vi "NIFPGA-MCS.get scan status.vi"(0 "i ref in":refnum<vi>, 3 "ms timeout (10000)":i32=10000, 5 "error in (no error)":errorcluster) -> (14 "i ref out":refnum<vi>, 16 "scanFinished ?":bool, 17 "timed out":bool, 19 "error out":errorcluster)   [LabVIEW 2014, in "NIFPGA-MCS.lvlib"]
doc: "Checks, if the recording of data has been finished."
uses:
  NIFPGA-MCS.lvlib
  CSinstr.lib/NI-FPGA-MCS/target/target.state.ctl
  CSCore/CSApplicationBaseClasses/DeviceBase/DeviceBase.lvlib
  CSinstr.lib/NI-FPGA-MCS/host/instrumentDriver/NI-FPGA-MCS_Driver.lvlib
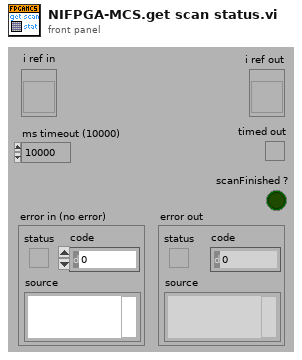
[diagram p1: front panel]
types:
  T1 = typedef "NIFPGA-MCS.lvlib/target.state.ctl" = enum16{"unknown", "configured", "triggerEnabled", "triggered", "done", "error"}
  T2 = typedef "NIFPGA-MCS.lvlib/NIFPGA-MCS.i attribute.ctl" = cluster{"fpgaViRef":T3}
  T3 = typedef "NI-FPGA-MCS_Driver.lvlib/fpga_vi_ref.ctl" = refnum<k20>
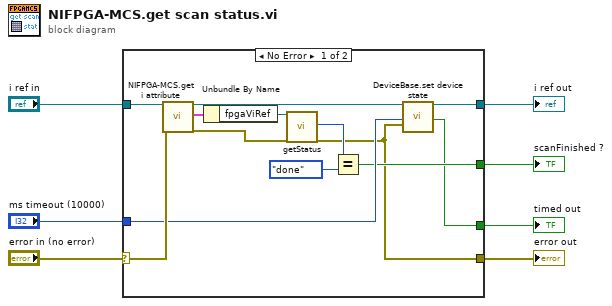
[diagram p0: block diagram]
diagram:
  n1 = case shown="No Error" "error in (no error)" {
    selector: "error in (no error)" -> [w19 w21]
    tunnel: "i ref in" -> [w20 w22]
    tunnel: [w16 w22] -> w5
    tunnel: [w8 w21] -> w4
    tunnel: "ms timeout (10000)" -> [w14 _]
    tunnel: [w9 _] -> w2
    tunnel: [w10 _] -> w1
    frame No Error {
      n2 = call "NIFPGA-MCS.get i attribute.vi"("i ref in"=w20, "error in (no error)"=w19) -> ("i ref out"=w13:refnum<vi>, "i attribute"=w17:T2, "error out"=w18:errorcluster)  [unwired: 15 in]
      n3 = Unbundle By Name(w17) -> ("fpgaViRef"=w15:T3)
      n4 = call "getStatus.vi"("fpga_vi_ref"=w15, "error in (no error)"=w18) -> ("state"=w12:T1, "error out"=w8:errorcluster)  [unwired: 15 in, 1 out]
      n5 = Equal?(x=w12, y=target.state."done") -> (x = y?=w10:bool)
      n6 = call "DeviceBase.set device state.vi"("i ref in"=w13, "ms timeout (10000)"=w14, "device error"=w8) -> ("i ref out"=w16:refnum<vi>, "timed out"=w9:bool)  [unwired: 14 in, 1 out]
    }
    frame Error {
    }
  }
  "error out" <- w4
  "i ref out" <- w5
  "timed out" <- w2
  "scanFinished ?" <- w1
